vi "Orion PDU Config Dialog.vi"(11 "Orion Parameters":T1) -> (2 "Cancelled?":bool, 3 "Orion Parameters out":T1)   [LabVIEW 2022 SP3, in "Orion PDU.lvclass"]
uses:
  Orion PDU.lvclass
  typedef Orion PDU Settings.ctl
panel:
  in  "Cancel Button":bool
  in  "OK Button":bool
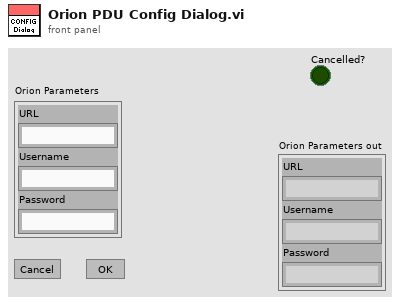
[diagram p1: front panel]
types:
  T1 = typedef "Orion PDU.lvclass/typedef Orion PDU Settings.ctl" = cluster{"URL":string, "Username":string, "Password":string}
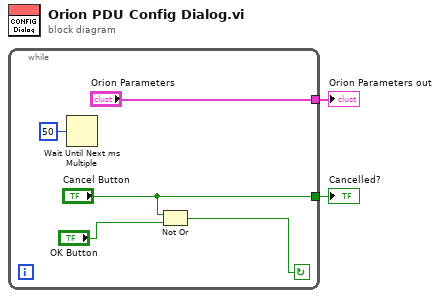
[diagram p0: block diagram]
diagram:
  n1 = while {
    tunnel: ["Orion Parameters"] -> w2
    tunnel: ["Cancel Button"] -> w1
    stop <- w5 continue-if-true
    n2 = Wait Until Next ms Multiple(millisecond multiple=u32 50) -> ()  [unwired: 1 out]
    n3 = Not Or(1:"OK Button", 2:"Cancel Button") -> (0:w5:bool)
  }
  "Orion Parameters out" <- w2
  "Cancelled?" <- w1
